vi "Write ServerRequest.vi"(10 "ServerRequest":refnum<queue>, 11 "TCPConnectionHandler in":refnum<class "TCPConnectionHandler.lvclass">) -> (3 "TCPConnectionHandler out":refnum<class "TCPConnectionHandler.lvclass">)   [LabVIEW 2013, in "MQTT Server.lvlib" / "TCPConnectionHandler.lvclass"]
uses:
  TCPConnectionHandler.lvclass
  Server class/Request -- cluster.ctl
  Control Packets/ControlPacket/ControlPacket.lvclass
  Server class/Response -- cluster.ctl
  TCPConnectionHandler.lvclass/TCPConnectionHandler.ctl
  Server class/Server.lvclass
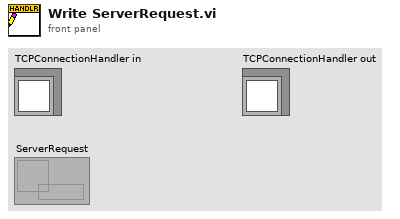
[diagram p1: front panel]
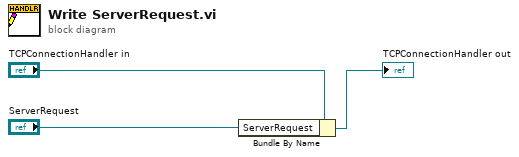
[diagram p0: block diagram]
diagram:
  n1 = Bundle By Name(cluster="TCPConnectionHandler in", "ServerRequest"="ServerRequest") -> (→"TCPConnectionHandler out":refnum<class "TCPConnectionHandler.lvclass">)
